vi "SA_SET_CF.vi"(4 "Send OPC? (T)":bool=TRUE, 5 "IsPSA(t)":bool, 6 "READ ONLY (T)":bool, 7 "Delay  (ms)":i64=1 caption="Delay Time (s)", 8 "error in":errorcluster {"code" format="%.0x"}, 9 "Freq Units":u16(ring)=1 items=["Hz", "MHz", "GHz"], 10 "SET CF ()":dbl, 11 "Session In":refnum<visa-resource-name>="GPIB0::18::INSTR") -> (0 "error out":errorcluster {"code" format="%.0x"}, 2 "READ CF ()":string, 3 "Session Out":refnum<visa-resource-name>)   [LabVIEW 2018]
uses:
  Initialize References/Station References Global.vi
  Keysight N9010A/Agilent MXA Series/Agilent MXA Series.lvlib
panel:
  out "RD(CMD)":string="FREQ:RF:CENT?"
  out "WR(CMD)":string
  in  "Timeout":u32=3000
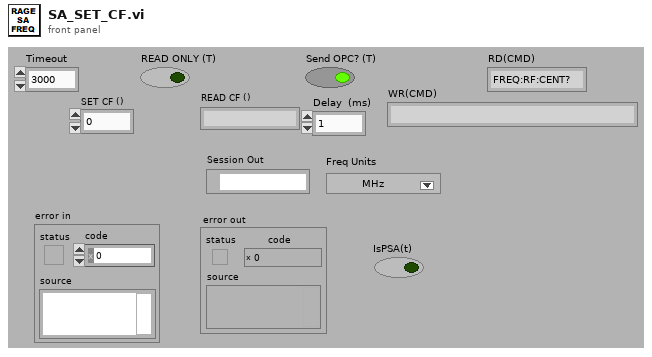
[diagram p1: front panel]
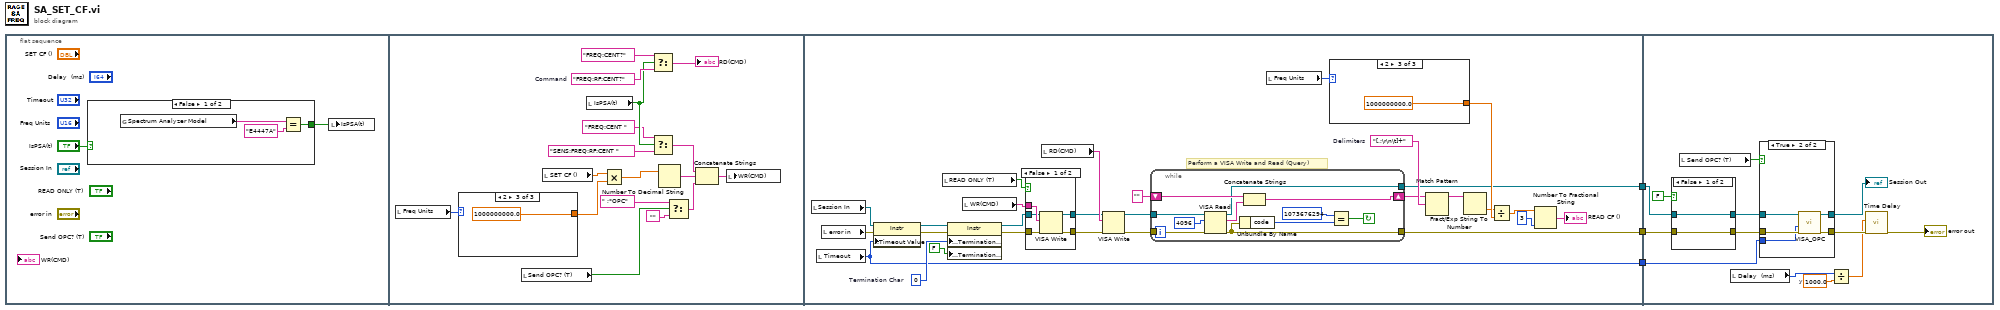
[diagram p0: block diagram]
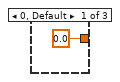
[diagram p3: hidden frame]
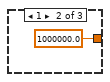
[diagram p4: hidden frame]
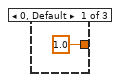
[diagram p5: hidden frame]
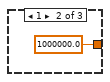
[diagram p6: hidden frame]
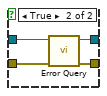
[diagram p9: hidden frame]
diagram:
  n1 = flat-sequence {
    tunnel: [w33] -> w3
    tunnel: [w32] -> w2
    tunnel: [w31] -> w1
    tunnel: w3 -> [w82]
    tunnel: w2 -> [w80]
    tunnel: w1 -> [w79]
    frame #0 {
      n2 = case shown="False" "IsPSA(t)" {
        selector: "IsPSA(t)" -> [_ w9]
        tunnel: [w6 w9] -> w5
        frame False {
          n3 = global read "Station References Global.vi" "Spectrum Analyzer Model"() -> (w8:string)
          n4 = Equal?(x=w8, y="E4447A") -> (x = y?=w6:bool)
        }
        frame True {
        }
      }
      n5 = local write "IsPSA(t)"(w5) -> ()
    }
    frame #1 {
      w17 = "FREQ:RF:CENT?"  # Command
      n6 = local read "Freq Units"() -> (w25:u16)
      n7 = case shown="2" w25 {
        tunnel: [0.0 ("y") 1000000.0 ("y") 1000000000.0 ("y")] -> w22
        frame 0, Default {
        }
        frame 1 {
        }
        frame 2 {
        }
      }
      n8 = local read "Send OPC? (T)"() -> (w10:bool)
      n9 = local read "SET CF ()"() -> (w24:dbl)
      n10 = local read "IsPSA(t)"() -> (w16:bool)
      n11 = Multiply(x=w24, y=w22) -> (x*y=w23:dbl)
      n12 = Select(t="FREQ:CENT?", s=w16, f=w17) -> (s? t:f=→"RD(CMD)":string)
      n13 = Select(t="FREQ:CENT ", s=w16, f="SENS:FREQ:RF:CENT " ("staticText")) -> (s? t:f=w19:string)
      n14 = Number To Decimal String(number=w23) -> (decimal integer string=w21:string)  [unwired: 1 in]
      n15 = Select(t=" ;*OPC" ("staticText"), s=w10, f="") -> (s? t:f=w13:string)
      n16 = Concatenate Strings(w19, w21, w13) -> (w26:string)
      n17 = local write "WR(CMD)"(w26) -> ()
    }
    frame #2 {
      w37 = "[,;\r\n\t]+"  # Delimiters
      w35 = u8 0  # Termination Char
      # "Perform a VISA Write and Read (Query)"
      n18 = local read "Session In"() -> (w53:refnum<visa-resource-name>)
      n19 = local read "Timeout"() -> (w33:u32)
      n20 = local read "error in"() -> (w55:errorcluster)
      n21 = property class="Instr"(reference=w53, error in=w55, "General Settings:Timeout Value"=w33) -> (reference out=w41:refnum<visa-resource-name>, error out=w39:errorcluster)
      n22 = local read "READ ONLY (T)"() -> (w54:bool)
      n23 = property class="Instr"(reference=w41, error in=w39, "Message Based Settings:Termination Character"=w35, "Message Based Settings:Termination Character Enable"=FALSE ("enable")) -> (reference out=w45:refnum<visa-resource-name>, error out=w40:errorcluster)
      n24 = local read "WR(CMD)"() -> (w56:string)
      n25 = case shown="False" w54 {
        tunnel: w40 -> [w65 w66]
        tunnel: [w64 w66] -> w42
        tunnel: w56 -> [w63 _]
        tunnel: w45 -> [w62 w67]
        tunnel: [w61 w67] -> w46
        frame False {
          n26 = VISA Write(VISA resource name=w62, write buffer=w63, error in (no error)=w65) -> (VISA resource name out=w61:refnum<visa-resource-name>, error out=w64:errorcluster)  [unwired: 1 out]
        }
        frame True {
        }
      }
      n27 = local read "RD(CMD)"() -> (w57:string)
      n28 = VISA Write(VISA resource name=w46, write buffer=w57, error in (no error)=w42) -> (VISA resource name out=w43:refnum<visa-resource-name>, error out=w44:errorcluster)  [unwired: 1 out]
      n29 = while {
        tunnel: w43 -> [w75]
        shift-right: [w69] -> w30
        shift-left: "" -> [w74]
        tunnel: w44 -> [w72]
        tunnel: [w71] -> w31
        tunnel: [w68] -> w32
        stop <- w70 continue-if-true
        n30 = VISA Read(VISA resource name=w75, byte count=u32 4096 ("byte count (0)"), error in (no error)=w72) -> (VISA resource name out=w68:refnum<visa-resource-name>, read buffer=w73:string, error out=w71:errorcluster)  [unwired: 1 out]
        n31 = Unbundle By Name(w71) -> ("code"=w77:i32)
        n32 = Concatenate Strings(w74, w73) -> (w69:string)
        n33 = Equal?(x=1073676294, y=w77) -> (x = y?=w70:bool)
      }
      n34 = local read "Freq Units"() -> (w52:u16)
      n35 = case shown="2" w52 {
        tunnel: [1.0 ("y") 1000000.0 ("y") 1000000000.0 ("y")] -> w49
        frame 0, Default {
        }
        frame 1 {
        }
        frame 2 {
        }
      }
      n36 = Match Pattern(string=w30, regular expression=w37) -> (before substring=w47:string)  [unwired: 4 out]
      n37 = Fract/Exp String To Number(string=w47) -> (number=w48:dbl)  [unwired: 3 in, 1 out]
      n38 = Divide(x=w48, y=w49) -> (x/y=w50:dbl)
      n39 = Number To Fractional String(number=w50, precision (6)=i16 3) -> (F-format string=→"READ CF ()":string)  [unwired: 2 in]
    }
    frame #3 {
      w83 = 1000.0  # y
      n40 = case shown="False" FALSE {
        tunnel: w80 -> [w99 w104]
        tunnel: [w99 w103] -> w90
        tunnel: w79 -> [w100 w102]
        tunnel: [w100 w101] -> w91
        frame False {
        }
        frame True {
          n41 = call "Error Query.vi"("error in (no error)"=w102, "VISA resource name"=w104) -> ("error out"=w101:errorcluster, "VISA resource name out"=w103:refnum<visa-resource-name>)  [unwired: 6 in, 2 out]
        }
      }
      n42 = local read "Send OPC? (T)"() -> (w84:bool)
      n43 = local read "Delay  (ms)"() -> (w85:i64)
      n44 = case shown="True" w84 {
        tunnel: w91 -> [w92 w98]
        tunnel: w90 -> [w93 w97]
        tunnel: [w93 w96] -> w89
        tunnel: [w92 w95] -> w88
        tunnel: w82 -> [_ w94]
        frame False {
        }
        frame True {
          n45 = call "VISA_OPC.vi"("error in"=w98, "Timeout"=w94, "Session In"=w97) -> ("error out"=w95:errorcluster, "Session Out"=w96:refnum<visa-resource-name>)  [unwired: 6 in, 1 out]
        }
      }
      "Session Out" <- w89
      n46 = Divide(x=w85, y=w83) -> (x/y=w86:dbl)
      n47 = call "Time Delay"("error in (no error)"=w88, "Delay Time (s)"=w86) -> ("error out"=→"error out":errorcluster)  [unwired: 9 in]
    }
  }
